vi "PDE Flexible Element_Boundary.vi"(2 "data":variant, 3 "y":dbl, 4 "x":dbl) -> (0 "error out":errorcluster, 1 "F(x, y)":dbl)   [LabVIEW 2023]
doc: "This VI implements the boundary condition."
panel:
  # "This is an example of a VI that the PDE solver can call by reference. All VIs called by the PDE solver must have the same connector pane."
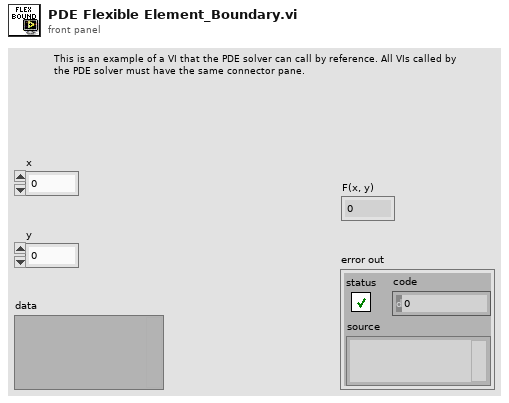
[diagram p1: front panel]
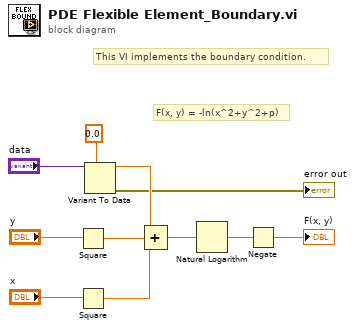
[diagram p0: block diagram]
diagram:
  # "This VI implements the boundary condition."
  # "F(x, y) = -ln(x^2+y^2+p)"
  n1 = Square(x="y") -> (x^2=w6:dbl)
  n2 = Square(x="x") -> (x^2=w5:dbl)
  n3 = Variant To Data(type=0.0, Variant="data") -> (data=w7:dbl, error out=→"error out":errorcluster)  [unwired: 1 in]
  n4 = Compound Arithmetic op=ADD(w7, w6, w5) -> (w4:dbl)
  n5 = Natural Logarithm(1:w4) -> (0:w3:dbl)
  n6 = Negate(x=w3) -> (-x=→"F(x, y)":dbl)
